vi "GASDAQ.vi"() -> ()   [LabVIEW 2013]
uses:
  <vilib>/Analysis/Matrix/NI_Matrix.lvlib
  old builds/Auto_DAQ/Auto_DAQ/AutoDAQ.exe/builds/DAQexe/Control 2.ctl
  <vilib>/Analysis/NI_AALPro.lvlib
  <vilib>/Utility/file.llb/Write Delimited Spreadsheet (string).vi
  <vilib>/Analysis/Matrix/Numeric/Conversions/Array To Matrix - RA2.vi
  <vilib>/DAQmx/create/channels.llb/DAQmx Create Channel (AI-Voltage-Basic).vi
  <vilib>/DAQmx/read.llb/DAQmx Read (Analog 1D DBL NChan 1Samp).vi
panel:
  in  "Auto-Update Name":bool
  out "DP vs. Flow Rate":cluster{"all rows":dbl[], "all rows":dbl[]}[](graph)
  out "Flow Rate vs. DP":cluster{"X":dbl[], "Y":dbl[]}[](graph)
  in  "SLPM Plot Multiplier":dbl=10.0 min=0.0 max=100.0 step=5.0 format="%#_13g"
  out "Flow Rate vs. DP":cluster{"all rows":dbl[], "all rows":dbl[]}[](graph)
  in  "Compare Data     flow_sampname.csv":path[](array[path])
  in  "Burst Fractions":bool
  in  "Burst Plot Max Press. (bar)":dbl=110.0
  in  "Baseline Data (optional)":path[](array[path])
  in  "Index Offset":dbl=1.0
  out "Countdown":dbl
  in  "Start Delay (s)":u32=2 max=10 step=1
  in  "# of Samples":dbl=1000.0
  in  "Infinite Sampling":bool=TRUE
  in  "Append to File":bool=TRUE
  out "Downstream":dbl
  out "Flow":dbl
  out "Upstream":dbl
  in  "Full Scale Flow (SLPM)":dbl=2.0
  in  "Max downstream (bar)":dbl=5.5
  in  "Max upstream (bar)":dbl=110.0
  in  "Sampling Delay (s)":dbl(knob)=1.0 min=0.0 max=60.0 step=0.25 scale=0.0..60.0
  out "Flow (SLPM)":dbl format="%_4f"
  out "Downstream (bar)":dbl format="%.2f"
  out "Upstream (bar)":dbl format="%.1f"
  in  "DAQ channels  GASDAQ/ai[Up]:[Flow]":tag="GASDAQ/ai0:2"
  out "Remaining Time":u32 format="%<%H:%M:%S>t"
  out "Last Meas.":string caption="Last Meas. (16)"
  in  "Sample Name":string="pretest"
  in  "Stop":bool
  out "Progress":i32(slide) max=300 scale=-1.0..9999.0
  in  "Working Directory":path=path "C:/National Instruments Downloads"
  out "Data Preview":string[][](table)
  in  "Flag":bool
  out "Acquired Data":T1(graph)
  # "Before you start:\n    •Turn on power supply, check DAQ channels\n    •Choose directory & sample name\n    •Adjust sample delay, plot options\n    •Begin pretest"
  # "Safety Glasses Recommended\n for high pressure measurements"
  # "Signal Settings"
  # "Acquired Data"
  # "Select 'Browse...' for multiple channels"
  # "Scaling:"
  # "Scale Factors"
  # "Last Build (v3.1): 4/25/2016 • Chris Williams"
  # "Remove/Reset files: Right Click > Data Operations"
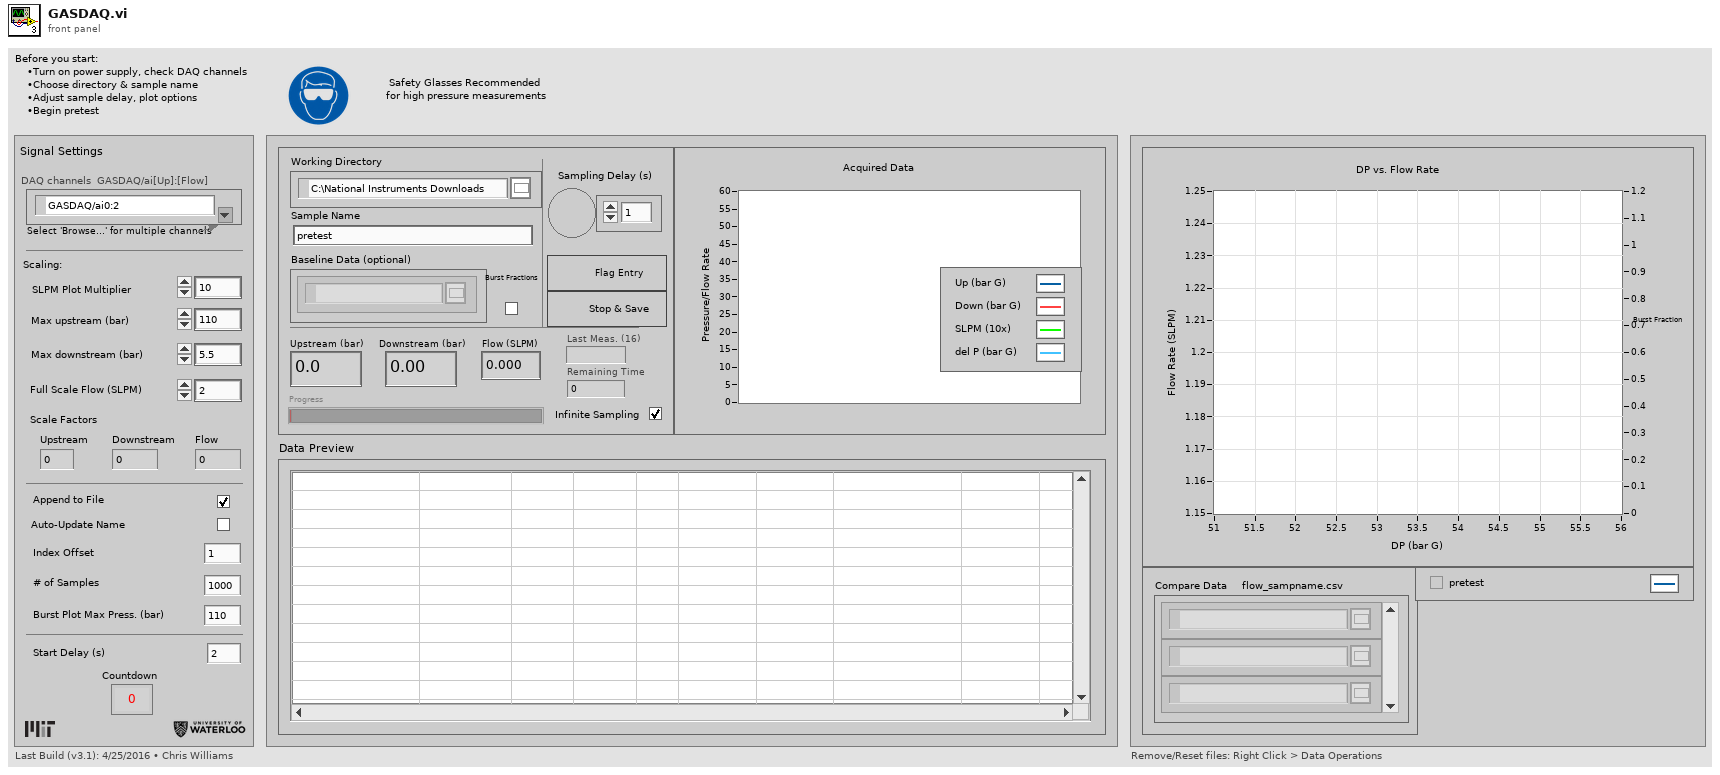
[diagram p1: front panel]
types:
  T1 = cluster{"data[0]":dbl, "data[1]":dbl, "data[2]":dbl, dbl}
  T2 = cluster{"data[0]":dbl, "data[1]":dbl, "data[2]":dbl, dbl}[]
  T3 = enum8{"Enabled", "Disabled", "Disabled and Grayed Out"}
  T4 = typedef "Control 2.ctl" = i32
  T5 = cluster{"data[0]":dbl, "data[1]":dbl, "data[2]":dbl}
  T6 = typedef "NI_Matrix.lvlib/RealMatrix.ctl" = dbl[][]
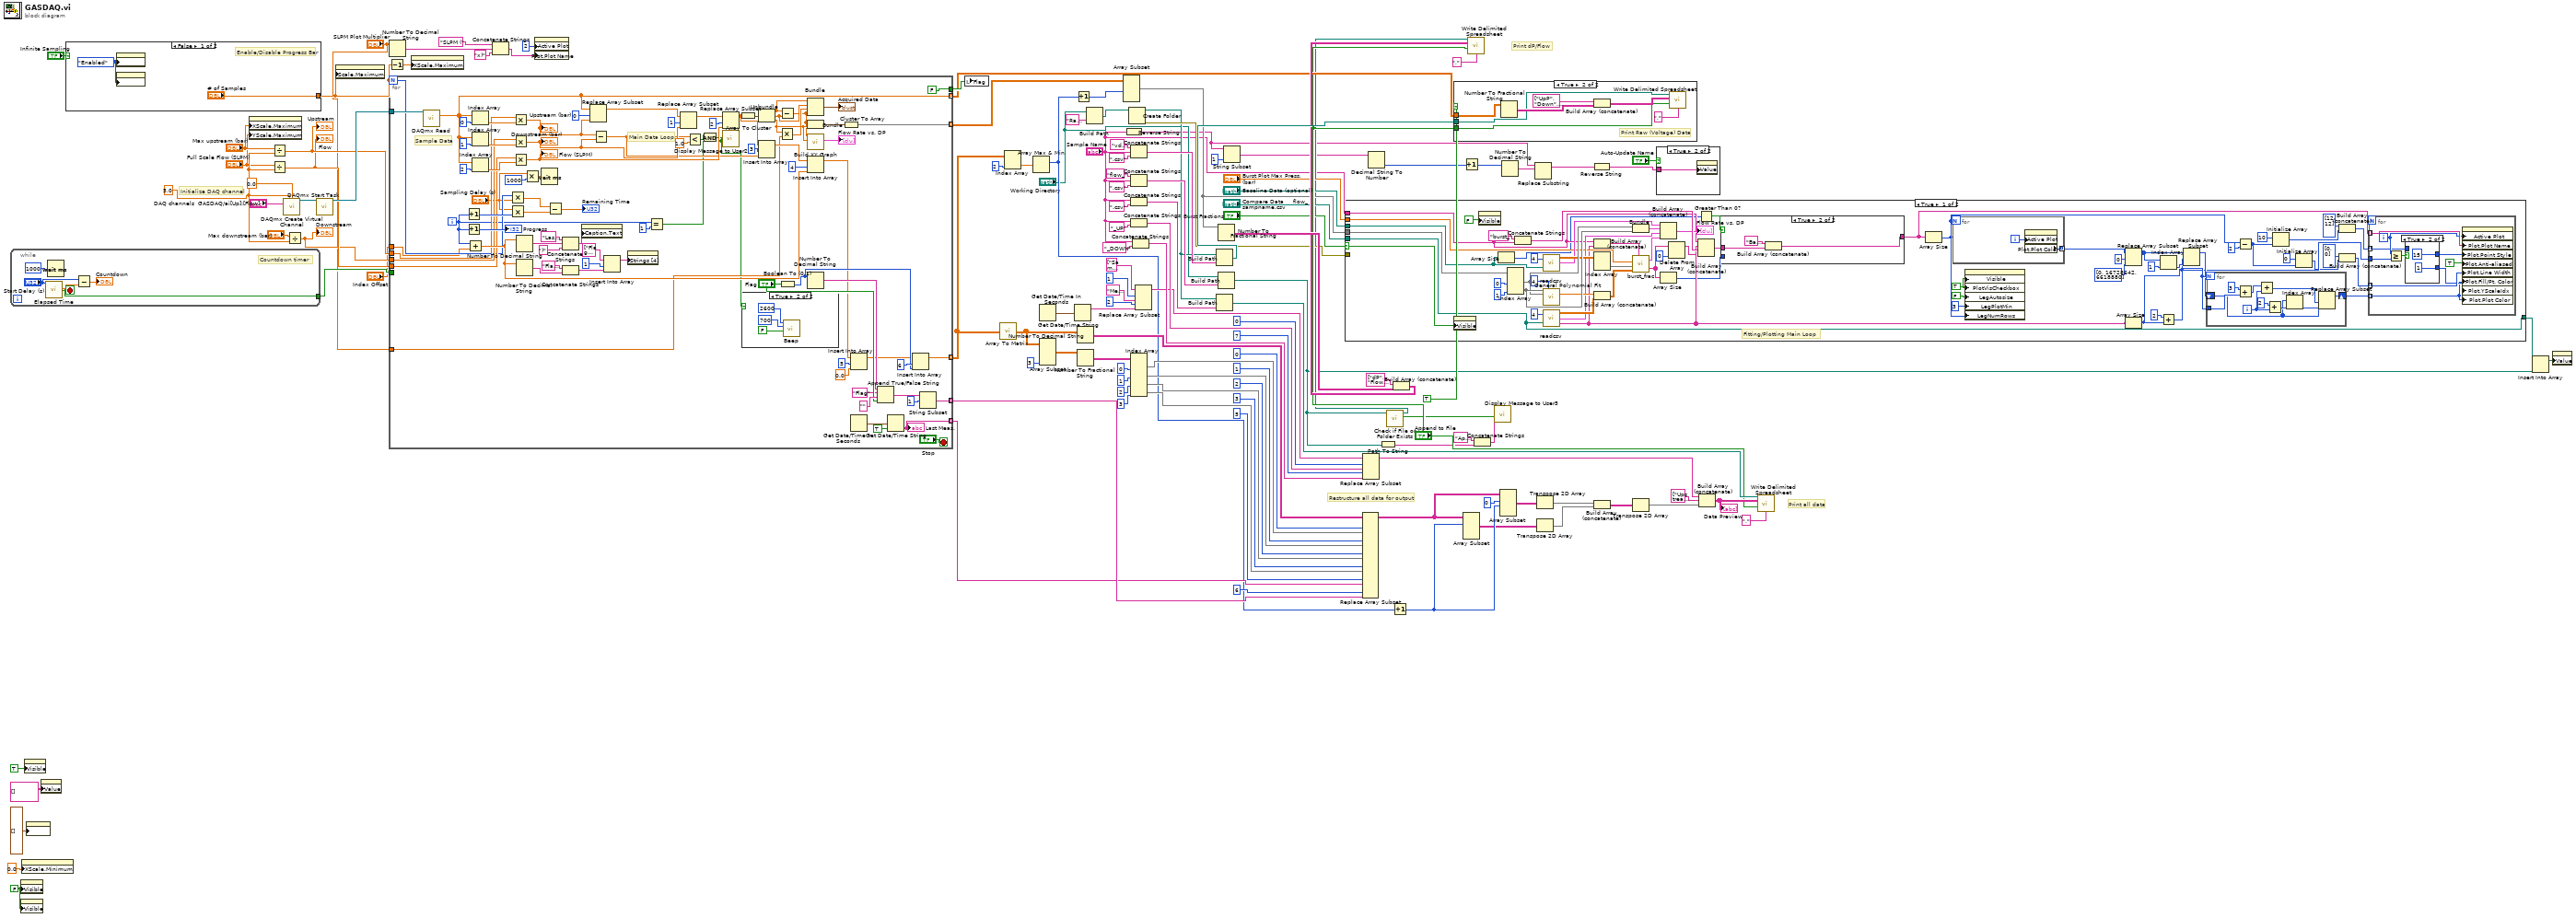
[diagram p0: block diagram]
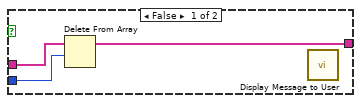
[diagram p3: hidden frame]
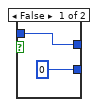
[diagram p4: hidden frame]
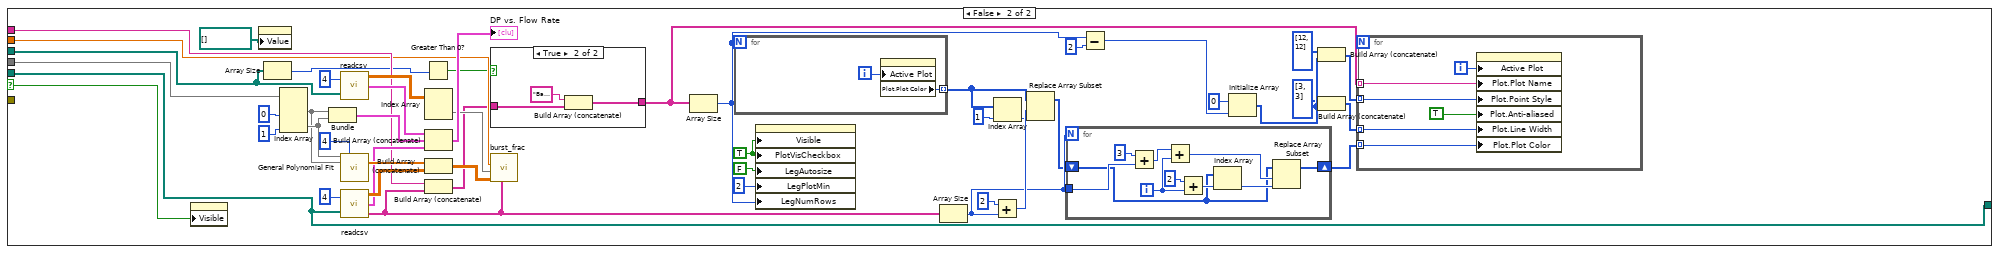
[diagram p5: hidden frame]
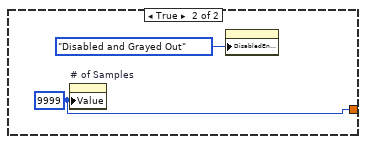
[diagram p8: hidden frame]
diagram:
  w22 = FALSE ("Visible")
  w60 = 5.0 ("maximum value")
  # "Restructure all data for output"
  # "Print dP/Flow"
  # "Print all data"
  # "Initialize DAQ channel"
  n1 = while {
    tunnel: [w129] -> w59
    stop <- w129 stop-if-true
    # "Countdown timer"
    n2 = call "Elapsed Time"("Time Target (s)"="Start Delay (s)") -> ("Elapsed Time (s)"=w131:dbl, "Time has Elapsed"=w129:bool)  [unwired: 11 in, 6 out]
    n3 = Wait (ms)(milliseconds to wait=u32 1000) -> ()  [unwired: 1 out]
    n4 = Subtract(x="Start Delay (s)", y=w131) -> (x-y=→"Countdown":dbl)
  }
  n5 = property on="Flow Rate vs. DP" class="XYGraph (strict)"("Visible"=w22) -> ()  [unwired: 2 in, 2 out]
  n6 = property on="DP vs. Flow Rate" class="XYGraph (strict)"("Visible"=w22) -> ()  [unwired: 2 in, 2 out]
  n7 = property on="Acquired Data" class="WFChart (strict)"("XScale.Minimum"=0.0 ("X Scale.Range:Minimum")) -> ()  [unwired: 2 in, 2 out]
  n8 = property on="Flow Rate vs. DP" class="XYGraph (strict)"("Visible"=TRUE) -> ()  [unwired: 2 in, 2 out]
  n9 = property on="Acquired Data" class="WFChart (strict)"("History Data"=T2 []) -> ()  [unwired: 2 in, 2 out]
  n10 = property on="Data Preview" class="Tbl (strict)"("Value"=string[][] [] ("Data Preview")) -> ()  [unwired: 2 in, 2 out]
  n11 = case shown="False" "Infinite Sampling" {
    tunnel: ["# of Samples" w134] -> w73
    frame False {
      w132 = T3."Enabled" ("Disabled")
      # "Enable/Disable Progress Bar"
      n12 = property on="# of Samples" class="DigNum (strict)"("DisabledEnum"=w132) -> ()  [unwired: 2 in, 2 out]
      n13 = property on="Progress" class="Slide (strict)"("DisabledEnum"=w132) -> ()  [unwired: 2 in, 2 out]
    }
    frame True {
      w134 = T4 9999 ("# of Meas.")
      n14 = property on="# of Samples" class="DigNum (strict)"("Value"=w134) -> ()  [unwired: 2 in, 2 out]
      n15 = property on="Progress" class="Slide (strict)"("DisabledEnum"=T3."Disabled and Grayed Out" ("Disabled")) -> ()  [unwired: 2 in, 2 out]
    }
  }
  n16 = property on="Flow Rate vs. DP" class="XYGraph (strict)"("XScale.Maximum"="Max upstream (bar)", "YScale.Maximum"="Full Scale Flow (SLPM)") -> ()  [unwired: 2 in, 2 out]
  n17 = Divide(x="Max upstream (bar)", y=w60) -> (x/y=w67:dbl)
  "Upstream" <- w67
  n18 = Divide(x="Full Scale Flow (SLPM)", y=w60) -> (x/y=w65:dbl)
  "Flow" <- w65
  n19 = call-poly <vilib>:"DAQmx Create Virtual Channel.vi"("maximum value"=w60, "minimum value"=0.0, "physical channels"="DAQ channels  GASDAQ/ai[Up]:[Flow]") -> ("task out"=w70:refnum<k21>)  [unwired: 11 in, 1 out]
  n20 = Divide(x="Max downstream (bar)", y=w60) -> (x/y=w63:dbl)
  "Downstream" <- w63
  n21 = call <vilib>:"DAQmx Start Task.vi"("task/channels in"=w70) -> ("task out"=w68:refnum<k21>)  [unwired: 13 in, 1 out]
  n22 = property on="Progress" class="Slide (strict)"("Scale.Maximum"=w73) -> ()  [unwired: 2 in, 2 out]
  n23 = Decrement(x=w73) -> (x-1=w72:dbl)
  n24 = Number To Decimal String(number="SLPM Plot Multiplier") -> (decimal integer string=w29:string)  [unwired: 1 in]
  n25 = for {
    N: w73 -> [w152]
    tunnel: [w209] -> w75 mode=indexing
    tunnel: [w202] -> w79 mode=indexing
    tunnel: [w193] -> w78 mode=indexing
    tunnel: [FALSE ("Flag")] -> w74
    tunnel: [w163] -> w41 mode=indexing
    tunnel: "Index Offset" -> [w150]
    tunnel: w68 -> [w156]
    tunnel: w67 -> [w155]
    tunnel: w63 -> [w154]
    tunnel: w65 -> [w153]
    tunnel: [w148] -> w38 mode=indexing
    tunnel: w59 -> [_]
    tunnel: "SLPM Plot Multiplier" -> [w143]
    i -> [w139]
    stop <- "Stop" stop-if-true
    # "Main Data Loop"
    # "Sample Data"
    n26 = call-poly <vilib>:"DAQmx Read.vi"("task/channels in"=w156) -> ("data"=w163:dbl[])  [unwired: 12 in, 2 out]
    n27 = Increment(x=w139) -> (x+1=w168:i32)
    n28 = Increment(x=w139) -> (x+1=→"Progress":i32)
    n29 = Add(x=w139, y=w150) -> (x+y=w179:dbl)
    n30 = Index Array(array=w163, index=0) -> (element=w176:dbl)
    n31 = Index Array(array=w163, index=1) -> (element=w175:dbl)
    n32 = Index Array(array=w163, index=2) -> (element=w161:dbl)
    n33 = Multiply(x=w152, y="Sampling Delay (s)") -> (x*y=w191:dbl)
    n34 = Multiply(x="Sampling Delay (s)", y=w168) -> (x*y=w169:dbl)
    n35 = Multiply(x=w155, y=w176) -> (x*y=w174:dbl)
    "Upstream (bar)" <- w174
    n36 = Multiply(x=w154, y=w175) -> (x*y=w172:dbl)
    "Downstream (bar)" <- w172
    n37 = Multiply(x=w153, y=w161) -> (x*y=w158:dbl)
    "Flow (SLPM)" <- w158
    n38 = Number To Decimal String(number=w179) -> (decimal integer string=w182:string)  [unwired: 1 in]
    n39 = Number To Decimal String(number=w179) -> (decimal integer string=w186:string)  [unwired: 1 in]
    n40 = Multiply(x="Sampling Delay (s)", y=u32 1000) -> (x*y=w199:dbl)
    n41 = Wait (ms)(milliseconds to wait=w199) -> ()  [unwired: 1 out]
    n42 = Subtract(x=w191, y=w169) -> (x-y=→"Remaining Time":dbl)
    n43 = Concatenate Strings("Flagged #" ("new element/subarray"), w186) -> (w184:string)
    n44 = Concatenate Strings("Last Meas. (" ("string"), w182, ")" ("string")) -> (w180:string)
    n45 = property on="Last Meas." class="Str"("Caption.Text"=w180) -> ()  [unwired: 2 in, 2 out]
    n46 = Replace Array Subset(array=w163, new element=w174, index=0) -> (w173:dbl[])
    n47 = Subtract(x=w174, y=w172) -> (x-y=w142:dbl)
    n48 = Insert Into Array(array=string[] ["Flag Entry"] ("Strings [4]"), index=1, new element=w184) -> (w185:string[])
    n49 = property on="Flag" class="Bool (strict)"("Strings [4]"=w185) -> ()  [unwired: 2 in, 2 out]
    n50 = Equal?(x=w139, y=1) -> (x = y?=w137:bool)
    n51 = Replace Array Subset(array=w173, new element=w172, index=1) -> (w160:dbl[])
    n52 = Less?(x=w142, y=1.0) -> (x < y?=w141:bool)
    n53 = And(x=w137, y=w141) -> (x .and. y?=w136:bool)
    n54 = Replace Array Subset(array=w160, new element=w158, index=2) -> (w159:dbl[])
    n55 = call "Display Message to User2"("Enable"=w136) -> ()  [unwired: 9 in, 2 out]
    n56 = Array To Cluster(array=w159) -> (cluster=w167:T5)
    n57 = case shown="True" w136 {
      frame False {
      }
      frame True {
        n58 = call <vilib>:"Beep.vi"("use system alert? (T)"=FALSE, "duration (msec)"=u32 700, "frequency (Hz)"=u32 2600) -> ()  [unwired: 9 in]
      }
    }
    n59 = Unbundle(w167) -> ("data[0]"=w166:dbl, "data[1]"=w165:dbl, "data[2]"=w146:dbl)
    n60 = Insert Into Array(array=w159, index=3, new element=w142) -> (w213:dbl[])
    n61 = Multiply(x=w146, y=w143) -> (x*y=w149:dbl)
    n62 = Subtract(x=w166, y=w165) -> (x-y=w145:dbl)
    n63 = Boolean To (0,1)(Boolean="Flag") -> (0, 1=w208:i16)
    n64 = Bundle("data[0]"=w166, "data[1]"=w165, w149, w145) -> (→"Acquired Data":cluster{"data[0]":dbl, "data[1]":dbl, dbl, dbl})  [unwired: 1 in]
    n65 = Bundle(w145, "data[2]"=w146) -> (w147:cluster{dbl, "data[2]":dbl})  [unwired: 1 in]
    n66 = call "Build XY Graph"("Y Input"=w146, "X Input"=w145) -> ("XY Graph"=→"Flow Rate vs. DP":cluster{"X":dbl[], "Y":dbl[]}[])  [unwired: 8 in, 1 out]
    n67 = Insert Into Array(array=w213, index=4, new element=w179) -> (w178:dbl[])
    n68 = Number To Decimal String(number=w208) -> (decimal integer string=w207:string)  [unwired: 1 in]
    n69 = Cluster To Array(cluster=w147) -> (array=w148:dbl[])
    n70 = Get Date/Time In Seconds() -> (seconds since 1Jan1904=w194:timestamp)
    n71 = Insert Into Array(array=w178, index=5, new element=0.0 ("new element/subarray")) -> (w196:dbl[])
    n72 = Append True/False String(1:"Flag", 2:"" ("false string"), 3:"Flag" ("true string"), 4:w207) -> (0:w203:string)
    n73 = Get Date/Time String(seconds (now)=w194, want seconds? (F)=TRUE) -> (time string=w193:string)  [unwired: 1 in, 1 out]
    "Last Meas." <- w193
    n74 = Insert Into Array(array=w196, index=6, new element=w208) -> (w209:dbl[])
    n75 = String Subset(string=w203, offset (0)=1) -> (substring=w202:string)  [unwired: 1 in]
  }
  n76 = property on="Acquired Data" class="WFChart (strict)"("XScale.Maximum"=w72) -> ()  [unwired: 2 in, 2 out]
  n77 = Concatenate Strings("SLPM (" ("string"), w29, "x)" ("Plot.Plot Name")) -> (w28:string)
  n78 = property on="Acquired Data" class="WFChart (strict)"("Active Plot"=u32 2, "Plot.Plot Name"=w28) -> ()  [unwired: 2 in, 2 out]
  n79 = local write "Flag"(w74) -> ()
  n80 = call-poly <vilib>:"Array To Matrix.vi"("Real 2D Array"=w75) -> ("Real Matrix"=w120:T6)
  n81 = Index Array(array=w75, index (col)=2 ("disabled index (col)")) -> (element=w124:dbl[])  [unwired: 1 in]
  n82 = Array Max & Min(array=w124) -> (max index (indices)=w37:i32)  [unwired: 3 out]
  n83 = Get Date/Time In Seconds() -> (seconds since 1Jan1904=w90:timestamp)
  n84 = Array Subset ("Get Submatrix")(array=w120, length (col)=3 ("column N")) -> (w121:T6)  [unwired: 3 in]
  n85 = Get Date/Time String(seconds (now)=w90) -> (date string=w77:string)  [unwired: 2 in, 1 out]
  n86 = Increment(x=w37) -> (x+1=w36:i32)
  n87 = Number To Decimal String(number=w120) -> (decimal integer string=w123:string[][])  [unwired: 1 in]
  n88 = Number To Fractional String(number=w121) -> (F-format string=w119:string[][])  [unwired: 3 in]
  n89 = Build Path(base path="Working Directory", name or relative path="Raw Data" ("new element/subarray")) -> (appended path=w51:path)
  n90 = Array Subset(array=w38, length (row)=w36) -> (w27:dbl[][])  [unwired: 3 in]
  n91 = Reverse String(1:"Sample Name") -> (0:w2:string)
  n92 = Create Folder(path (use dialog)=w51) -> (created path=w19:path, error out=w21:errorcluster)  [unwired: 2 in, 1 out]
  n93 = Index Array(array=w119, index (col) #1=0 ("disabled index (col)"), index (col) #2=1 ("index (col)"), index (col) #3=2 ("index (col)"), index (col) #4=3 ("index (col)")) -> (element #1=w115:string[], element #2=w114:string[], element #3=w113:string[], element #4=w111:string[])  [unwired: 4 in]
  n94 = Concatenate Strings("vdata_" ("string"), "Sample Name", ".csv" ("string")) -> (w50:string)
  n95 = Concatenate Strings("flow_" ("string"), "Sample Name", ".csv" ("string")) -> (w46:string)
  n96 = Concatenate Strings("Sample Name", ".csv" ("string")) -> (w48:string)
  n97 = Concatenate Strings("Sample Name", "_UP" ("string")) -> (w87:string)
  n98 = Concatenate Strings("Sample Name", "_DOWN" ("string")) -> (w85:string)
  n99 = Replace Array Subset(array=string[] ["Sample Name", "", "", "", "", "", "", "Sample name", ""], new element #1="Measured:  " ("string"), index #1=1 ("index"), new element #2=w77, index #2=2 ("index")) -> (w82:string[])
  n100 = Build Path(base path=w19, name or relative path=w50) -> (appended path=w49:path)
  n101 = Build Path(base path=w19, name or relative path=w48) -> (appended path=w47:path)
  n102 = Number To Fractional String(number=w27) -> (F-format string=w45:string[][])  [unwired: 3 in]
  n103 = Build Path(base path="Working Directory", name or relative path=w46) -> (appended path=w4:path)
  n104 = String Subset(string=w2, length (rest)=1 ("length (rest)")) -> (substring=w6:string)  [unwired: 1 in]
  n105 = case shown="True" "Burst Fractions" {
    selector: "Burst Fractions" -> [w243 w321]
    tunnel: w27 -> [w279 w359]
    tunnel: "Sample Name" -> [w240 w342]
    tunnel: "Baseline Data (optional)" -> [w230 w316]
    tunnel: "Burst Plot Max Press. (bar)" -> [w242 w320]
    tunnel: "Compare Data     flow_sampname.csv" -> [w223 w313]
    tunnel: w21 -> [_ _]
    tunnel: [w223 w313] -> w5
    frame True {
      w262 = TRUE ("Visible")
      # "Fitting/Plotting Main Loop"
      n106 = property on="Flow Rate vs. DP" class="XYGraph (strict)"("Visible"=w243) -> ()  [unwired: 2 in, 2 out]
      n107 = property on="Flow Rate vs. DP" class="XYGraph (strict)"("Visible"=FALSE) -> ()  [unwired: 2 in, 2 out]
      n108 = Array Size(array=w230) -> (size(s)=w231:i32)
      n109 = Index Array(array=w279, index (col) #1=0 ("disabled index (col)"), index (col) #2=1 ("index (col)")) -> (element #1=w276:dbl[], element #2=w277:dbl[])  [unwired: 2 in]
      n110 = Concatenate Strings("burst_" ("array"), w240) -> (w266:string)
      n111 = call "readcsv.vi"("Order"=4, "Baseline Data (optional)"=w230) -> ("B(x)"=w275:dbl[][], "Array"=w261:cluster{"all rows":dbl[], "all rows":dbl[]}[])  [unwired: 1 out]
      n112 = call <vilib>:"General Polynomial Fit.vi"("Y"=w277, "polynomial order"=4, "X"=w276) -> ("Polynomial Coefficients"=w268:dbl[])  [unwired: 9 in, 3 out]
      n113 = call "readcsv.vi"("Order"=4, "Baseline Data (optional)"=w223) -> ("B(x)"=w274:dbl[][], "Array"=w265:cluster{"all rows":dbl[], "all rows":dbl[]}[], "Names"=w239:string[])
      n114 = Build Array (concatenate)(w240, w239) -> (w238:string[])
      n115 = Index Array(array=w275) -> (element=w269:dbl[])  [unwired: 2 in]
      n116 = Build Array (concatenate)(w268, w274) -> (w270:dbl[][])
      n117 = Bundle(w276, w277) -> (w260:cluster{dbl[], dbl[]})  [unwired: 1 in]
      n118 = call "burst_frac.vi"("Upper Pressure"=w242, "B(x)"=w269, "Gs(x)"=w270, "Names"=w238) -> ("Array"=w264:cluster{"Ramp Pattern":dbl[], "Array":dbl[]}[], "Frac Names"=w225:string[])  [unwired: 1 in]
      n119 = Build Array (concatenate)(w261, w260, w265, w264) -> (→"Flow Rate vs. DP":cluster{"Ramp Pattern":dbl[], "Array":dbl[]}[])
      n120 = Array Size(array=w225) -> (size(s)=w226:i32)
      n121 = Delete From Array(array=w225, index=0) -> (array with subset deleted=w227:string[])  [unwired: 1 in, 1 out]
      n122 = Greater Than 0?(x=w231) -> (x > 0?=w232:bool)
      n123 = Build Array (concatenate)(w240, w239, w266, w227) -> (w229:string[])
      n124 = case shown="True" w232 {
        tunnel: [w282 w284] -> w228
        tunnel: w229 -> [w283 w285]
        tunnel: w226 -> [w281 _]
        frame False {
          n125 = Delete From Array(array=w283, length=w281) -> (array with subset deleted=w282:string[])  [unwired: 1 in, 1 out]
          n126 = call "Display Message to User"() -> ()  [unwired: 10 in, 2 out]
        }
        frame True {
          n127 = Build Array (concatenate)("Baseline" ("Plot.Plot Name"), w285) -> (w284:string[])
        }
      }
      n128 = Array Size(array=w228) -> (size(s)=w244:i32)
      n129 = for {
        N: w244 -> [_]
        tunnel: [w298] -> w236 mode=indexing
        i -> [w297]
        n130 = property on="Flow Rate vs. DP" class="XYGraph (strict)"("Active Plot"=w297) -> ("Plot.Plot Color"=w298:u32)  [unwired: 2 in, 2 out]
      }
      n131 = property on="Flow Rate vs. DP" class="XYGraph (strict)"("Visible"=w262, "PlotVisCheckbox"=w262, "LegAutosize"=FALSE, "LegPlotMin"=u32 3 ("Legend:Plot Minimum"), "LegNumRows"=w244) -> ()  [unwired: 2 in, 2 out]
      n132 = Replace Array Subset(array=w236, new element=u32[] [0, 16728642, 6618880] ("new element/subarray"), index=0) -> (w235:u32[])
      n133 = Array Size(array=w239) -> (size(s)=w247:i32)
      n134 = Index Array(array=w235, index=1) -> (element=w248:u32)
      n135 = Add(x=2, y=w247) -> (x+y=w224:i32)
      n136 = Replace Array Subset(array=w235, new element=w248, index=w224) -> (w246:u32[])
      n137 = for {
        N: w247 -> [_]
        tunnel: w247 -> [w292]
        shift-right: [w288] -> w245
        shift-left: w246 -> [w287]
        i -> [w290]
        n138 = Add(x=3, y=w292) -> (x+y=w291:i32)
        n139 = Add(x=w291, y=w290) -> (x+y=w289:i32)
        n140 = Add(x=2, y=w290) -> (x+y=w295:i32)
        n141 = Index Array(array=w287, index=w295) -> (element=w294:u32)
        n142 = Replace Array Subset(array=w287, new element=w294, index=w289) -> (w288:u32[])
      }
      n143 = Subtract(x=w244, y=2) -> (x-y=w221:i32)
      n144 = Initialize Array(u8 10 ("Plot.Line Width"), w221) -> (w254:u8[])
      n145 = Initialize Array(u8 0 ("element"), w221) -> (w220:u8[])
      n146 = Build Array (concatenate)(u8[] [12, 12] ("Plot.Point Style"), w254) -> (w253:u8[])
      n147 = Build Array (concatenate)(u8[] [0, 0] ("Plot.Point Style"), w220) -> (w256:u8[])
      n148 = for {
        tunnel: w228 -> [w308] mode=indexing
        tunnel: w253 -> [w301] mode=indexing
        tunnel: w256 -> [w307] mode=indexing
        tunnel: w245 -> [w299] mode=indexing
        tunnel: w224 -> [w304]
        i -> [w305]
        n149 = Greater Or Equal?(x=w305, y=w304) -> (x >= y?=w303:bool)
        n150 = case shown="True" w303 {
          tunnel: [0 ("x") 1 ("x")] -> w302
          tunnel: w301 -> [w309 _]
          tunnel: [w309 15 ("x")] -> w300
          frame False {
          }
          frame True {
          }
        }
        n151 = property on="Flow Rate vs. DP" class="XYGraph (strict)"("Active Plot"=w305, "Plot.Plot Name"=w308, "Plot.Point Style"=w300, "Plot.Anti-aliased"=TRUE, "Plot.Line Width"=w307, "Plot.Fill/Pt. Color"=w299, "Plot.YScaleIdx"=w302, "Plot.Plot Color"=w299) -> ()  [unwired: 2 in, 2 out]
      }
    }
    frame False {
      w345 = TRUE ("Visible")
      n152 = property on="DP vs. Flow Rate" class="XYGraph (strict)"("Visible"=w321) -> ()  [unwired: 2 in, 2 out]
      n153 = property on="Compare Data     flow_sampname.csv" class="Arr (strict)"("Value"=path[] [] ("Compare Data (flow/base_samp.csv)")) -> ()  [unwired: 2 in, 2 out]
      n154 = Array Size(array=w316) -> (size(s)=w318:i32)
      n155 = Index Array(array=w359, index (col) #1=0 ("disabled index (col)"), index (col) #2=1 ("index (col)")) -> (element #1=w355:dbl[], element #2=w356:dbl[])  [unwired: 2 in]
      n156 = Bundle(w355, w356) -> (w343:cluster{dbl[], dbl[]})  [unwired: 1 in]
      n157 = call "readcsv.vi"("Order"=4, "Baseline Data (optional)"=w316) -> ("B(x)"=w354:dbl[][], "Array"=w344:cluster{"all rows":dbl[], "all rows":dbl[]}[])  [unwired: 1 out]
      n158 = call <vilib>:"General Polynomial Fit.vi"("Y"=w356, "polynomial order"=4, "X"=w355) -> ("Polynomial Coefficients"=w347:dbl[])  [unwired: 9 in, 3 out]
      n159 = call "readcsv.vi"("Order"=4, "Baseline Data (optional)"=w313) -> ("B(x)"=w353:dbl[][], "Array"=w346:cluster{"all rows":dbl[], "all rows":dbl[]}[], "Names"=w322:string[])
      n160 = Greater Than 0?(x=w318) -> (x > 0?=w317:bool)
      n161 = Index Array(array=w354) -> (element=w348:dbl[])  [unwired: 2 in]
      n162 = Build Array (concatenate)(w344, w343, w346) -> (→"DP vs. Flow Rate":cluster{"all rows":dbl[], "all rows":dbl[]}[])
      n163 = Build Array (concatenate)(w347, w353) -> (w349:dbl[][])
      n164 = Build Array (concatenate)(w342, w322) -> (w315:string[])
      n165 = case shown="True" w317 {
        tunnel: w315 -> [w361 w364]
        tunnel: [w361 w362] -> w314
        frame False {
        }
        frame True {
          n166 = Build Array (concatenate)("Baseline" ("Plot.Plot Name"), w364) -> (w362:string[])
        }
      }
      n167 = call "burst_frac.vi"("Upper Pressure"=w320, "B(x)"=w348, "Gs(x)"=w349, "Names"=w322) -> ()  [unwired: 1 in, 2 out]
      n168 = Array Size(array=w314) -> (size(s)=w323:i32)
      n169 = for {
        N: w323 -> [_]
        tunnel: [w376] -> w331 mode=indexing
        i -> [w375]
        n170 = property on="DP vs. Flow Rate" class="XYGraph (strict)"("Active Plot"=w375) -> ("Plot.Plot Color"=w376:u32)  [unwired: 2 in, 2 out]
      }
      n171 = property on="DP vs. Flow Rate" class="XYGraph (strict)"("Visible"=w345, "PlotVisCheckbox"=w345, "LegAutosize"=FALSE, "LegPlotMin"=u32 2 ("Legend:Plot Minimum"), "LegNumRows"=w323) -> ()  [unwired: 2 in, 2 out]
      n172 = Array Size(array=w322) -> (size(s)=w326:i32)
      n173 = Add(x=2, y=w326) -> (x+y=w329:i32)
      n174 = Index Array(array=w331, index=1) -> (element=w327:u32)
      n175 = Replace Array Subset(array=w331, new element=w327, index=w329) -> (w325:u32[])
      n176 = for {
        N: w326 -> [_]
        tunnel: w326 -> [w370]
        shift-right: [w366] -> w324
        shift-left: w325 -> [w365]
        i -> [w368]
        n177 = Add(x=3, y=w370) -> (x+y=w369:i32)
        n178 = Add(x=w369, y=w368) -> (x+y=w367:i32)
        n179 = Add(x=2, y=w368) -> (x+y=w373:i32)
        n180 = Index Array(array=w365, index=w373) -> (element=w372:u32)
        n181 = Replace Array Subset(array=w365, new element=w372, index=w367) -> (w366:u32[])
      }
      n182 = Subtract(x=w323, y=2) -> (x-y=w338:i32)
      n183 = Initialize Array(u8 0 ("Plot.Line Width"), w338) -> (w335:u8[])
      n184 = Build Array (concatenate)(u8[] [12, 12] ("Plot.Point Style"), w335) -> (w334:u8[])
      n185 = Build Array (concatenate)(u8[] [3, 3] ("Plot.Point Style"), w335) -> (w337:u8[])
      n186 = for {
        tunnel: w314 -> [w382] mode=indexing
        tunnel: w334 -> [w380] mode=indexing
        tunnel: w337 -> [w379] mode=indexing
        tunnel: w324 -> [w377] mode=indexing
        i -> [w381]
        n187 = property on="DP vs. Flow Rate" class="XYGraph (strict)"("Active Plot"=w381, "Plot.Plot Name"=w382, "Plot.Point Style"=w380, "Plot.Anti-aliased"=TRUE, "Plot.Line Width"=w379, "Plot.Plot Color"=w377) -> ()  [unwired: 2 in, 2 out]
      }
    }
  }
  n188 = Replace Array Subset(array=w123, new element #1=w115, index (col) #1=0 ("disabled index (col)"), new element #2=w114, index (col) #2=1 ("index (col)"), new element #3=w113, index (col) #3=2 ("index (col)"), new element #4=w111, index (col) #4=3 ("index (col)"), new element #5=w78, index (col) #5=5 ("index (col)"), new element #6=w79, index (col) #6=6 ("index (col)")) -> (w104:string[][])  [unwired: 6 in]
  n189 = Replace Array Subset(array=w82, new element #1=w87, index #1=0 ("index"), new element #2=w85, index #2=7 ("index")) -> (w92:string[])
  n190 = Decimal String To Number(string=w6) -> (number=w13:i32)  [unwired: 2 in, 1 out]
  n191 = Path To String(path=w4) -> (string=w18:string)
  n192 = call <vilib>:"Check if File or Folder Exists.vi"("path"=w4) -> ("file or folder exists?"=w15:bool, "dup path"=w20:path)  [unwired: 8 in, 1 out]
  n193 = Increment(x=w37) -> (x+1=w103:i32)
  n194 = Build Array (concatenate)(string[] ["dP", "Flow Rate"], w45) -> (w43:string[][])
  n195 = case shown="True" TRUE ("Save voltage data") {
    tunnel: w49 -> [_ w383]
    tunnel: w41 -> [_ w386]
    tunnel: "Append to File" -> [_ w384]
    frame False {
    }
    frame True {
      # "Print Raw (Voltage) Data"
      n196 = Number To Fractional String(number=w386) -> (F-format string=w387:string[][])  [unwired: 3 in]
      n197 = Build Array (concatenate)(string[] ["UpP", "Down", "Flow"], w387) -> (w388:string[][])
      n198 = call-poly <vilib>:"Write Delimited Spreadsheet.vi"("file path (dialog if empty)"=w383, "2D data"=w388, "append to file? (new file:F)"=w384, "delimiter (\\t)"="," ("delimiter (\\t)")) -> ()  [unwired: 10 in, 2 out]
    }
  }
  n199 = Array Subset(array=w104, index (row)=w103) -> (w101:string[][])  [unwired: 3 in]
  n200 = Increment(x=w13) -> (x+1=w12:i32)
  n201 = call-poly <vilib>:"Write Delimited Spreadsheet.vi"("file path (dialog if empty)"=w20, "2D data"=w43, "append to file? (new file:F)"="Append to File", "delimiter (\\t)"="," ("delimiter (\\t)")) -> ()  [unwired: 10 in, 2 out]
  n202 = Concatenate Strings("Appending data to existing files in " ("delimiter (\\t)"), w18) -> (w16:string)
  n203 = call "Display Message to User3"("Enable"=w15, "Message"=w16) -> ()  [unwired: 8 in, 2 out]
  n204 = Array Subset(array=w104, index (row)=0 ("index"), length (row)=w103) -> (w102:string[][])  [unwired: 2 in]
  n205 = Number To Decimal String(number=w12) -> (decimal integer string=w11:string)  [unwired: 1 in]
  n206 = Replace Substring(4:w11, 5:w2) -> (1:w10:string)  [unwired: 2 in, 1 out]
  n207 = Transpose 2D Array(2D array=w102) -> (transposed array=w100:string[][])
  n208 = Transpose 2D Array(2D array=w101) -> (transposed array=w99:string[][])
  n209 = Reverse String(1:w10) -> (0:w7:string)
  n210 = Build Array (concatenate)(w100, w99) -> (w98:string[][])
  n211 = Transpose 2D Array(2D array=w98) -> (transposed array=w97:string[][])
  n212 = case shown="True" "Auto-Update Name" {
    tunnel: w7 -> [_ w390]
    frame False {
    }
    frame True {
      n213 = property on="Sample Name" class="Str"("Value"=w390) -> ()  [unwired: 2 in, 2 out]
    }
  }
  n214 = Build Array (concatenate)(w92, string[] ["Upstream (bar G)", "Down (bar G)", "SLPM", "del p (bar)", "Index", "Timestamp", "Flags", "Upstream", "Downstream", "SLPM", "del P", "Index", "Timestamp", "Flags"], w97) -> (w94:string[][])
  "Data Preview" <- w94
  n215 = call-poly <vilib>:"Write Delimited Spreadsheet.vi"("file path (dialog if empty)"=w47, "2D data"=w94, "append to file? (new file:F)"="Append to File", "delimiter (\\t)"="," ("delimiter (\\t)")) -> ()  [unwired: 10 in, 2 out]
  n216 = Insert Into Array(array=w5, new element=w4) -> (w3:path[])  [unwired: 1 in]
  n217 = property on="Compare Data     flow_sampname.csv" class="Arr (strict)"("Value"=w3) -> ()  [unwired: 2 in, 2 out]
